vi "lab 1.4.vi"() -> ()   [LabVIEW 2020]
uses:
  <vilib>/express/express analysis/Spectral/Block/exnSpectralBlock spectral measurements peak poly.vi
  <vilib>/express/express analysis/Spectral/Block/exnSpectralBlock spectral measurements peak WFM.vi
  <vilib>/express/express analysis/Spectral/XNode/ExpressSpectralMeasurementsBlockNode.xnode
  <vilib>/measure/NI_MABase.lvlib
panel:
  out "Waveform Graph 2":cluster{"f0":dbl, "df":dbl, "magnitude":dbl[]}(graph)
  out "Waveform Graph":waveform(dbl)(graph)
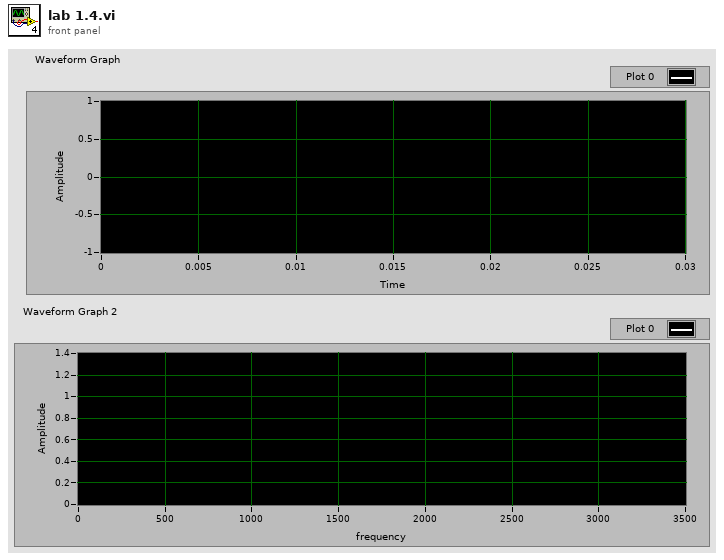
[diagram p1: front panel]
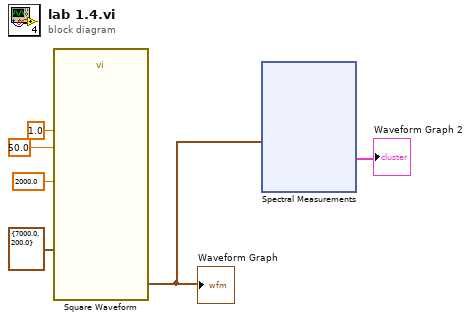
[diagram p0: block diagram]
diagram:
  n1 = call <vilib>:"Square Waveform.vi"("duty cycle (%)"=50.0, "sampling info"=cluster{"Fs":dbl, "#s":dbl} {"Fs"=7000.0, "#s"=200.0}, "amplitude"=1.0, "frequency"=2000.0) -> ("signal out"=w2:waveform(dbl))  [unwired: 6 in, 1 out]
  "Waveform Graph" <- w2
  n2 = xnode "Spectral Measurements"("Signals"=w2) -> ("FFT - (Peak)"=→"Waveform Graph 2":cluster{"f0":dbl, "df":dbl, "magnitude":dbl[]})  [unwired: 1 in, 2 out]
